vi "WaitForInputTrigger.vi"(8 "Error In":errorcluster, 10 "Trigger Input Configuration":T1={"Type"=enum."None", "Timeout (ms)"=100, "Delay (ms)"=0, "Digital IO Line (1-14)"=1, "Digital IO Mode"=enum."Falling"}, 11 "Kiethley 2602 In":refnum<visa-resource-name>) -> (0 "Error Out":errorcluster, 3 "Keithley 2602 Out":refnum<visa-resource-name>)   [LabVIEW 2012]
uses:
  TriggerInputConfiguration.ctl
  TriggerInputType.ctl
  driver/Public/Controls/TriggerMode.ctl
  libs/LV-Utilities/LV-Utilities.lvlib
  driver/Keithley-2602.lvlib
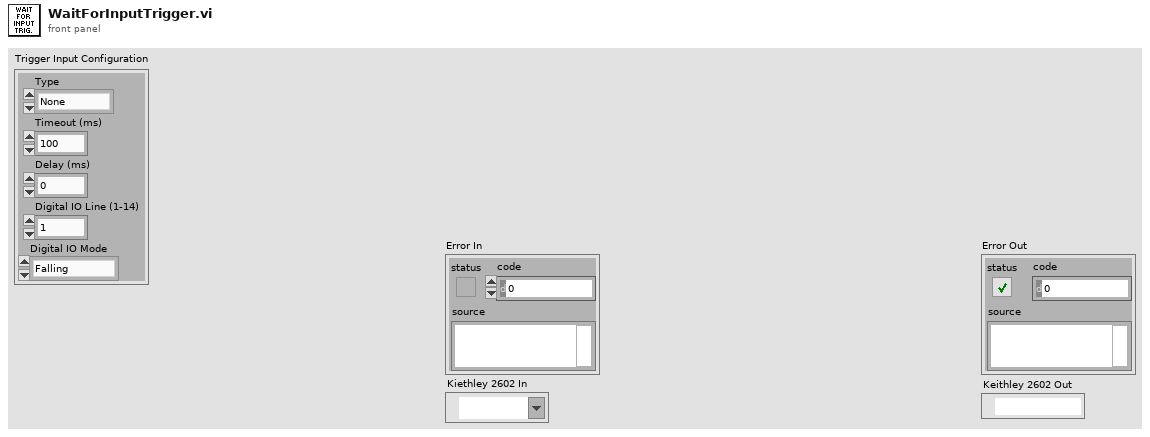
[diagram p1: front panel]
types:
  T1 = typedef "TriggerInputConfiguration.ctl" = cluster{"Type":T2, "Timeout (ms)":u32, "Delay (ms)":u32, "Digital IO Line (1-14)":u8, "Digital IO Mode":T3}
  T2 = typedef "TriggerInputType.ctl" = enum16{"None", "Digital IO", "Bus"}
  T3 = typedef "Keithley-2602.lvlib/TriggerMode.ctl" = enum16{"Falling", "Rising", "Either", "Synchronous"}
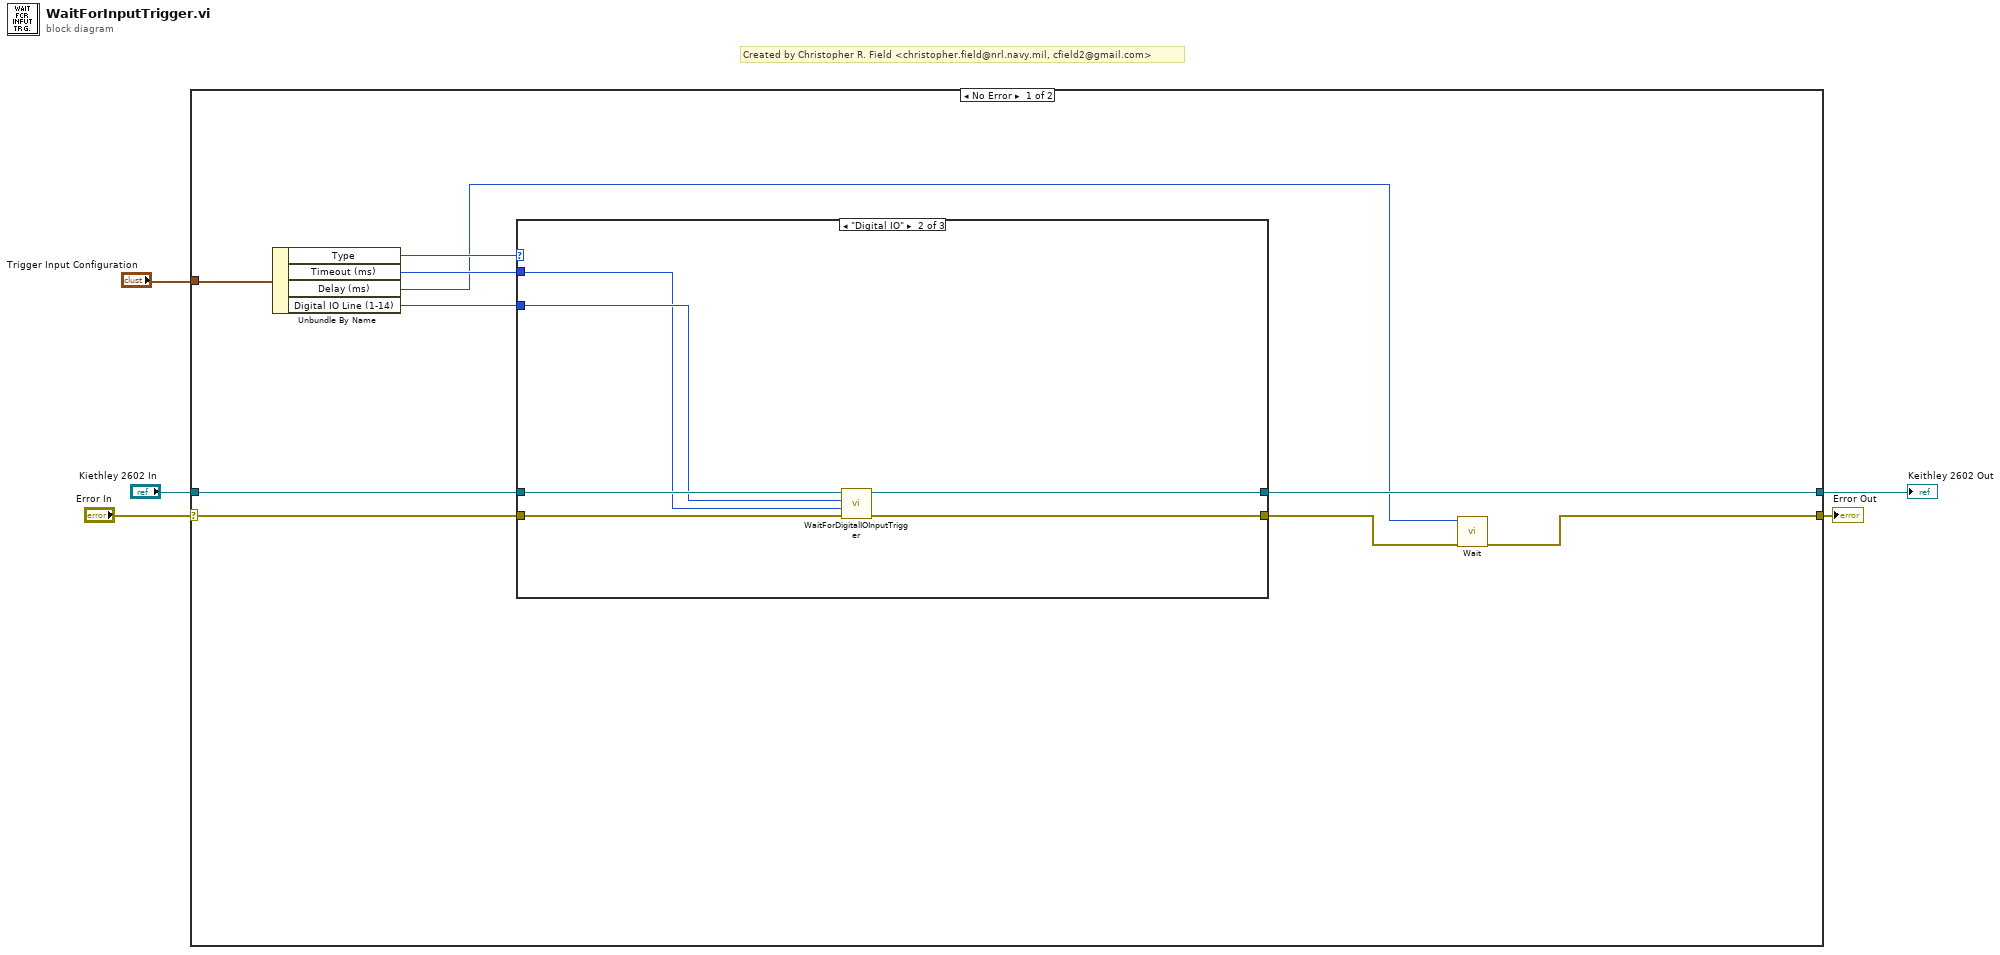
[diagram p0: block diagram]
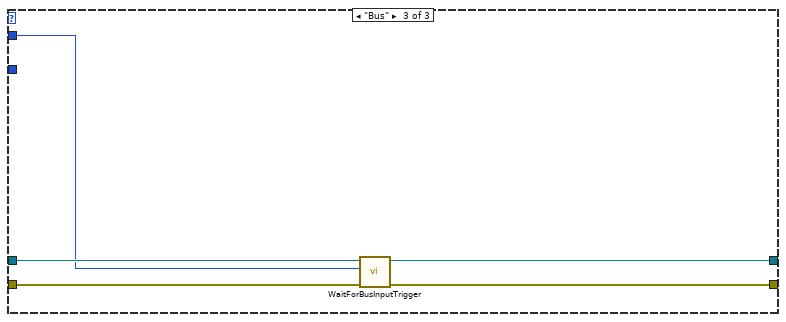
[diagram p3: hidden frame]
diagram:
  # "Created by Christopher R. Field <christopher.field@nrl.navy.mil, cfield2@gmail.com>"
  n1 = case shown="No Error" "Error In" {
    selector: "Error In" -> [w13 w30]
    tunnel: [w11 w30] -> w4
    tunnel: [w14 w29] -> w3
    tunnel: "Kiethley 2602 In" -> [w15 w29]
    tunnel: "Trigger Input Configuration" -> [w6 _]
    frame No Error {
      n2 = Unbundle By Name(w6) -> ("Type"=w10:T2, "Timeout (ms)"=w9:u32, "Delay (ms)"=w7:u32, "Digital IO Line (1-14)"=w8:u8)
      n3 = case shown="\"Digital IO\"" w10 {
        tunnel: w15 -> [w17 w23 w28]
        tunnel: [w17 w22 w25] -> w14
        tunnel: w13 -> [w16 w20 w27]
        tunnel: [w16 w21 w26] -> w12
        tunnel: w9 -> [_ w18 w24]
        tunnel: w8 -> [_ w19 _]
        frame "None", Default {
        }
        frame "Digital IO" {
          n4 = call "WaitForDigitalIOInputTrigger.vi"("Error In"=w20, "Timeout (ms)"=w18, "Line (1-14)"=w19, "Keithley 2602 In"=w23) -> ("Error Out"=w21:errorcluster, "Keithley 2602 Out"=w22:refnum<visa-resource-name>)  [unwired: 6 in]
        }
        frame "Bus" {
          n5 = call "WaitForBusInputTrigger.vi"("Error In"=w27, "Timeout (ms)"=w24, "Keithley 2602 In"=w28) -> ("Error Out"=w26:errorcluster, "Keithley 2602 Out"=w25:refnum<visa-resource-name>)  [unwired: 7 in]
        }
      }
      n6 = call "Wait.vi"("Error In"=w12, "Wait Time (msec)"=w7) -> ("Error Out"=w11:errorcluster)  [unwired: 9 in]
    }
    frame Error {
    }
  }
  "Error Out" <- w4
  "Keithley 2602 Out" <- w3
